vi "SwissSPAD Live_Settings Window.vi"() -> ()   [LabVIEW 2021]
uses:
  SwissSPAD Live_SS2 DAQ Parameters 3.ctl
  SwissSPAD Live_SS2 Gate Definition.ctl
  SwissSPAD Live_File Information.ctl
  SwissSPAD Live_Gate Characteristics.ctl
  SwissSPAD Live_Image ROI Information.ctl
  Phasor/Image Binning Options.ctl
  SwissSPAD Live_SSx PCB Version.ctl
  SwissSPAD Live_SS3 DAQ Parameters.ctl
  SwissSPAD Live_SS3 Gate Definition.ctl
  SS3 Gate Width Definition Mode.ctl
  SwissSPAD Live_SS3 Displayed Image v2.ctl
  SwissSPAD Live_Image Display Options.ctl
  SwissSPAD Live_FPGA Data to Display.ctl
  SwissSPAD Live_Settings Q Element.ctl
  SwissSPAD Live_Settings Q Action.ctl
  SwissSPAD Live_Gate Configuration Action.ctl
  SwissSPAD Live_Settings List.ctl
  SwissSPAD Live_SS2 Gate Configuration.ctl
  SwissSPAD Live_Q [Element].ctl
  SwissSPAD Live_Q Event List.ctl
  SwissSPAD Live_Globals.vi
  Variant/Variant to Data/Variant to Data.lvlib
panel:
  in  "Tab Control":T1(tab)
  in  "Top Half":bool
  in  "Bottom Half":bool
  out "Top Connected":bool caption="Connected"
  in  "Connect to Top FPGA":bool
  out "Top FPGA Serial Number":string
  out "Top Bitstream Version":string
  in  "Top Bitfile Path":path
  out "Bottom Connected":bool caption="Connected"
  in  "Connect to FPGA(s)":bool
  out "Detector PCB Version":T2
  out "Bottom FPGA Serial Number":string
  out "Bottom Bitstream Version":string
  in  "Bottom Bitfile Path":path
  in  "Auto Reset FPGA":bool
  in  "Microlens":bool
  in  "SS3 DAQ Parameters":T3={"10 bits"=FALSE, "# Exposure Sequences"=0, "# 1-bit Frame per Gate"=255, "Gate Shift"=0, "# Gate Pairs per Set"=0, "# Sets"=1, "Laser Period"=0.0, "Sync Period"=0.0, "Gate Offset"=0, "Auto-adjust Gate Offset"=FALSE, "Gate Definition"={"gs_psincdec_0"=0, "gs_psincdec_1"=0, "gs_no_shift_adj_1"=0, "gate_adj_2"=0}, "Gate Width (ns)"=0.0, "Reversed Shift"=FALSE, "Intensity Mode"=FALSE, "Gate Definition Mode"=enum."Item 0"} {"Gate Width (ns)" min=0.0 max=100.0 format="%#_5g"; "# Sets" min=1}
  in  "Buffer Size (# 8-bit Gates)":u32=1 min=1
  out "Gate Characteristics":T6 {"Gate Images Span" format="%#.3g"; "Gate Shift" format="%#.3g"; "Gate Image Exposure" format="%#.3g"; "Gate Image Integration" format="%#.3g"; "Predicted Gate Width" format="%#.3g"}
  in  "Preset Configuration":u16(ring) items=["User-defined configuration", "Gate Configuration 1", "Gate Configuration 2", "Gate Configuration 3", "Gate Configuration 4", "Gate Configuration 5", "Gate Configuration 6", "Gate Configuration 7"]
  in  "SS2 DAQ Parameters":T7={"10 bits"=FALSE, "# Exposure Sequences"=1, "# 1-bit Frame per Gate"=255, "Gate Shift"=0, "# Gates per Set"=1, "# Sets"=1, "Laser Period"=0.0, "Sync Period"=0.0, "Gate Offset"=0, "Auto-adjust Gate Offset"=FALSE, "Gate Definition"={"gs_psincdec_0"=0, "gs_psincdec_1"=0, "gs_psincdec_2"=0, "gs_psincdec_3"=0, "gs_no_shift_adj_1"=0, "gs_no_shift_adj_2"=0, "gs_no_shift_adj_3"=0}, "Reversed Shift"=FALSE} {"Sync Period" min=0.0 max=4.294967295 format="%#.3f"; "Laser Period" min=0.0 format="%#.3f"; "# 1-bit Frame per Gate" min=255 max=255; "# Sets" min=1; "# Gates per Set" min=1}
  in  "FPGA Data to Display":T9
  in  "Use Histogram Cursors":bool
  in  "SS3 Displayed Image":T10 caption="Image to Display"
  in  "Image Binning Options":T11={"Use Image Binning"=FALSE, "X Bin"=1, "Y Bin"=1} {"Y Bin" min=1; "X Bin" min=1}
  in  "Image ROI Information":T12
  in  "Image Display Options":T13={"Remove Screamers"=FALSE, "Delta"=0.0, "Equalize Histogram"=FALSE, "Percentile"=2.0, "Hot Pixel Mask Image"=path "", "Use Hot Pixel Mask"=FALSE} {"Percentile" min=0 max=100}
  in  "Save Sum of All Gates Preview":bool
  in  "SS3 Hot Pixel Mismatch Detection":bool
  in  "SS3 Gate Slip Correction":bool
  in  "Delay between Datasets":dbl[unit]
  in  "Scrambled File Flag":bool
  in  "# Datasets in Series":i32=1 min=1
  in  "File Information":T14={"File Folder"=path "", "File Name"="", "File Index"=0, "Author"="", "Sample"="", "Compression"=FALSE, "Compression Level"=9} {"Compression Level" max=9}
  in  "Histogram Bin Size":i32=256 min=1 step=1
  in  "Verbose Saving":bool
  in  "Verbose Settings":bool
  in  "Use Image Display Options":bool
  in  "Histogram Bins Number":i32=256 min=1 step=1
  # "Image Histogram"
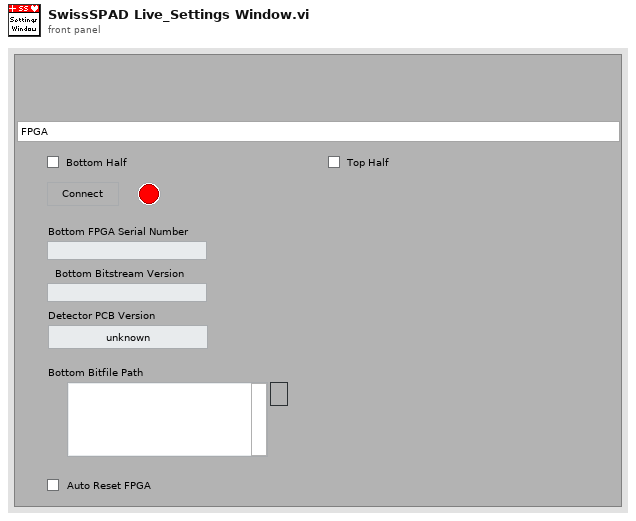
[diagram p1: front panel]
types:
  T1 = enum32{"FPGA", "Acquisition Parameters", "Image Parameters", "File Information", "UI Settings"}
  T2 = typedef "SwissSPAD Live_SSx PCB Version.ctl" = enum16{"unknown", "SS2 PCB1", "SS2 PCB2", "SS3 PCB1"}
  T3 = typedef "SwissSPAD Live_SS3 DAQ Parameters.ctl" = cluster{"10 bits":bool, "# Exposure Sequences":u32, "# 1-bit Frame per Gate":u32, "Gate Shift":u32, "# Gate Pairs per Set":u32, "# Sets":u32, "Laser Period":dbl[unit], "Sync Period":dbl[unit], "Gate Offset":u32, "Auto-adjust Gate Offset":bool, "Gate Definition":T4, "Gate Width (ns)":dbl, "Reversed Shift":bool, "Intensity Mode":bool, "Gate Definition Mode":T5}
  T4 = typedef "SwissSPAD Live_SS3 Gate Definition.ctl" = cluster{"gs_psincdec_0":u32, "gs_psincdec_1":u32, "gs_no_shift_adj_1":u32, "gate_adj_2":u32}
  T5 = typedef "SS3 Gate Width Definition Mode.ctl" = enum32{"Item 0", "Item 1"}
  T6 = typedef "SwissSPAD Live_Gate Characteristics.ctl" = cluster{"Predicted Gate Width":dbl[unit], "Gate Image Integration":dbl[unit], "Gate Image Exposure":dbl[unit], "Gate Shift":dbl[unit], "Gate Images Span":dbl[unit]}
  T7 = typedef "SwissSPAD Live_SS2 DAQ Parameters 3.ctl" = cluster{"10 bits":bool, "# Exposure Sequences":u32, "# 1-bit Frame per Gate":u32, "Gate Shift":u32, "# Gates per Set":u32, "# Sets":u32, "Laser Period":dbl[unit], "Sync Period":dbl[unit], "Gate Offset":u32, "Auto-adjust Gate Offset":bool, "Gate Definition":T8, "Reversed Shift":bool}
  T8 = typedef "SwissSPAD Live_SS2 Gate Definition.ctl" = cluster{"gs_psincdec_0":u32, "gs_psincdec_1":u32, "gs_psincdec_2":u32, "gs_psincdec_3":u32, "gs_no_shift_adj_1":u32, "gs_no_shift_adj_2":u32, "gs_no_shift_adj_3":u32}
  T9 = typedef "SwissSPAD Live_FPGA Data to Display.ctl" = enum16{"Bottom FPGA", "Top FPGA", "Both"}
  T10 = typedef "SwissSPAD Live_SS3 Displayed Image v2.ctl" = enum16{"G2 Gate", "INT Gate", "INT - G2"}
  T11 = typedef "Image Binning Options.ctl" = cluster{"Use Image Binning":bool, "X Bin":i32, "Y Bin":i32}
  T12 = typedef "SwissSPAD Live_Image ROI Information.ctl" = cluster{"Save ROI Only":bool, "Left":u16, "Top":u16, "Right":u16, "Bottom":u16, "Use Current ROI":bool}
  T13 = typedef "SwissSPAD Live_Image Display Options.ctl" = cluster{"Remove Screamers":bool, "Delta":sgl, "Equalize Histogram":bool, "Percentile":sgl, "Hot Pixel Mask Image":path, "Use Hot Pixel Mask":bool}
  T14 = typedef "SwissSPAD Live_File Information.ctl" = cluster{"File Folder":path, "File Name":string, "File Index":u32, "Author":string, "Sample":string, "Compression":bool, "Compression Level":u8}
  T15 = typedef "SwissSPAD Live_Settings Q Element.ctl" = cluster{"Action":T16, "Data":variant}
  T16 = typedef "SwissSPAD Live_Settings Q Action.ctl" = enum16{"Idle", "Initialization", "Refresh All Parameters", "Store Current Configuration", "Rename Current Configuration", "Delete Current Configuration", "Update Image ROI Information", "Load Hot Pixel Mask Image", "Quit"}
  T17 = cluster{"Connect to FPGA(s)":refnum<vi>, "Bottom Connected":refnum<vi>, "Preset Configuration":refnum<vi>, "SS2 DAQ Parameters":refnum<vi>, "SS3 DAQ Parameters":refnum<vi>, "SS3 Displayed Image":refnum<vi>, "Bottom FPGA Serial Number":refnum<vi>, "Detector PCB Version":refnum<vi>, "SS3 Gate Slip Correction":refnum<vi>, "Scrambled File Flag":refnum<vi>, "Top Connected":refnum<vi>, "Top FPGA Serial Number":refnum<vi>, "SS3 Hot Pixel Mismatch Detection":refnum<vi>}
  T18 = enum32{"Invalid", "Standard", "Closed", "Hidden", "Minimized", "Maximized"}
  T19 = typedef "SwissSPAD Live_Gate Configuration Action.ctl" = enum16{"Get Gate Configuration Name", "Get Configuration by Name", "Add Gate Configuration", "Delete Gate Configuration", "Rename Gate Configuration"}
  T20 = typedef "SwissSPAD Live_Settings List.ctl" = enum16{"FPGA:Bottom Half", "FPGA:Top Half", "FPGA:Bottom Bitfile Path", "FPGA:Top Bitfile Path", "FPGA:Bottom Bitstream Version", "FPGA:Top Bitstream Version", "FPGA:Auto Reset FPGA", "FPGA:Bottom FPGA Serial Number", "FPGA:Top FPGA Serial Number", "FPGA:Detector PCB Version", "Acquisition Parameters:Microlens", "Acquisition Parameters:SS2 DAQ Parameters", "Acquisition Parameters:Gate Configuration Array", "Acquisition Parameters:SS3 DAQ Parameters", "Acquisition Parameters:Buffer Size (# 8-bit Gates)", "File Information:File Information", "File Information:# Datasets in Series", "File Information:Scrambled File Flag", "File Information:SS3 Gate Slip Correction", "File Information:SS3 Hot Pixel Mismatch Detection", "File Information:Delay between Datasets", "File Information:Save Sum of All Gates Preview", "Image Parameters:Image ROI Information", "Image Parameters:Image Binning Options", "Image Parameters:SS3 Displayed Image", "Image Parameters:Image Display Options", "Image Parameters:Use Histogram Cursors", "Image Parameter:FPGA Data to Display", "UI Settings:Histogram Bins Number", "UI Settings:Histogram Bin Size", "UI Settings:Use Image Display Options", "UI Settings:Verbose Settings", "UI Settings:Verbose Saving"}
  T21 = typedef "SwissSPAD Live_Internal Variables.ctl" = cluster{"okCFrontPanelDevices Refnum":refnum<k24>, "Bottom Device Refnum":refnum<k24>, "Display Image":T22, "# Live Images":i32, "relative s":dbl, "# Image Sets":i32, "Message":string, "Current Image Set":i32, "# Datasets in Series":i32, "Current Dataset":i32, "Live Mode":bool, "Recording Mode":bool, "Record Button":refnum<vi>, "\nLive Button":refnum<vi>, "SwissSPAD Live Gate Image Data Q Name":string, "Discard First Image":bool, "Image Information":T12, "Image Binning Options":T11, "Bottom FPGA Serial Number":string, "Detector PCB Version":T2, "# Acquisitions":u32, "10 bits":bool, "Top FPGA Serial Number":string, "Top Device Refnum":refnum<k24>, "okCFrontPanel Refnum":refnum<k24>}
  T22 = typedef "IMAQ Image.ctl" = refnum<image>
  T23 = typedef "SwissSPAD Live_SS2 Gate Configuration.ctl" = cluster{"Gate Configuration":string, "Gate Offset":u32, "Gate Definition":T8}
  T24 = typedef "SwissSPAD Live_Q [Element].ctl" = cluster{"SwissSPAD Q Event":T25, "Data":variant}
  T25 = typedef "SwissSPAD Live_Q Event List.ctl" = enum16{"---- UI ----", "Idle", "Initialization", "Init FPGA(s)", "Init Top FPGA (deprecated)", "FPGA(s) Status", "Top FPGA Status (deprecated)", "Reset FPGA(s)", "Reset Top FPGA (deprecated)", "Refresh Display Image", "Quit", "---- DAQ ----", "Start Recording", "Start Live Acquisition", "Initialize Recording Mode", "Initialize FPGA (Live Mode)", "Get Image Set", "Get Single Image", "Update Image Display", "Stop Live Acquisition", "Stop Data Recording", "Stop Data Saving", "---- Image ----", "Copy Data to Clipboard", "Set Image Palette", "Save Displayed Image with Overlay", "Save Image Data as TIFF"}
  T26 = typedef "SS2 DAQ_Settings Window Messages.ctl" = enum16{"Idle", "Subscribe", "Unsubscribe", "Refresh Parameter", "Refresh All Parameters", "Quit"}
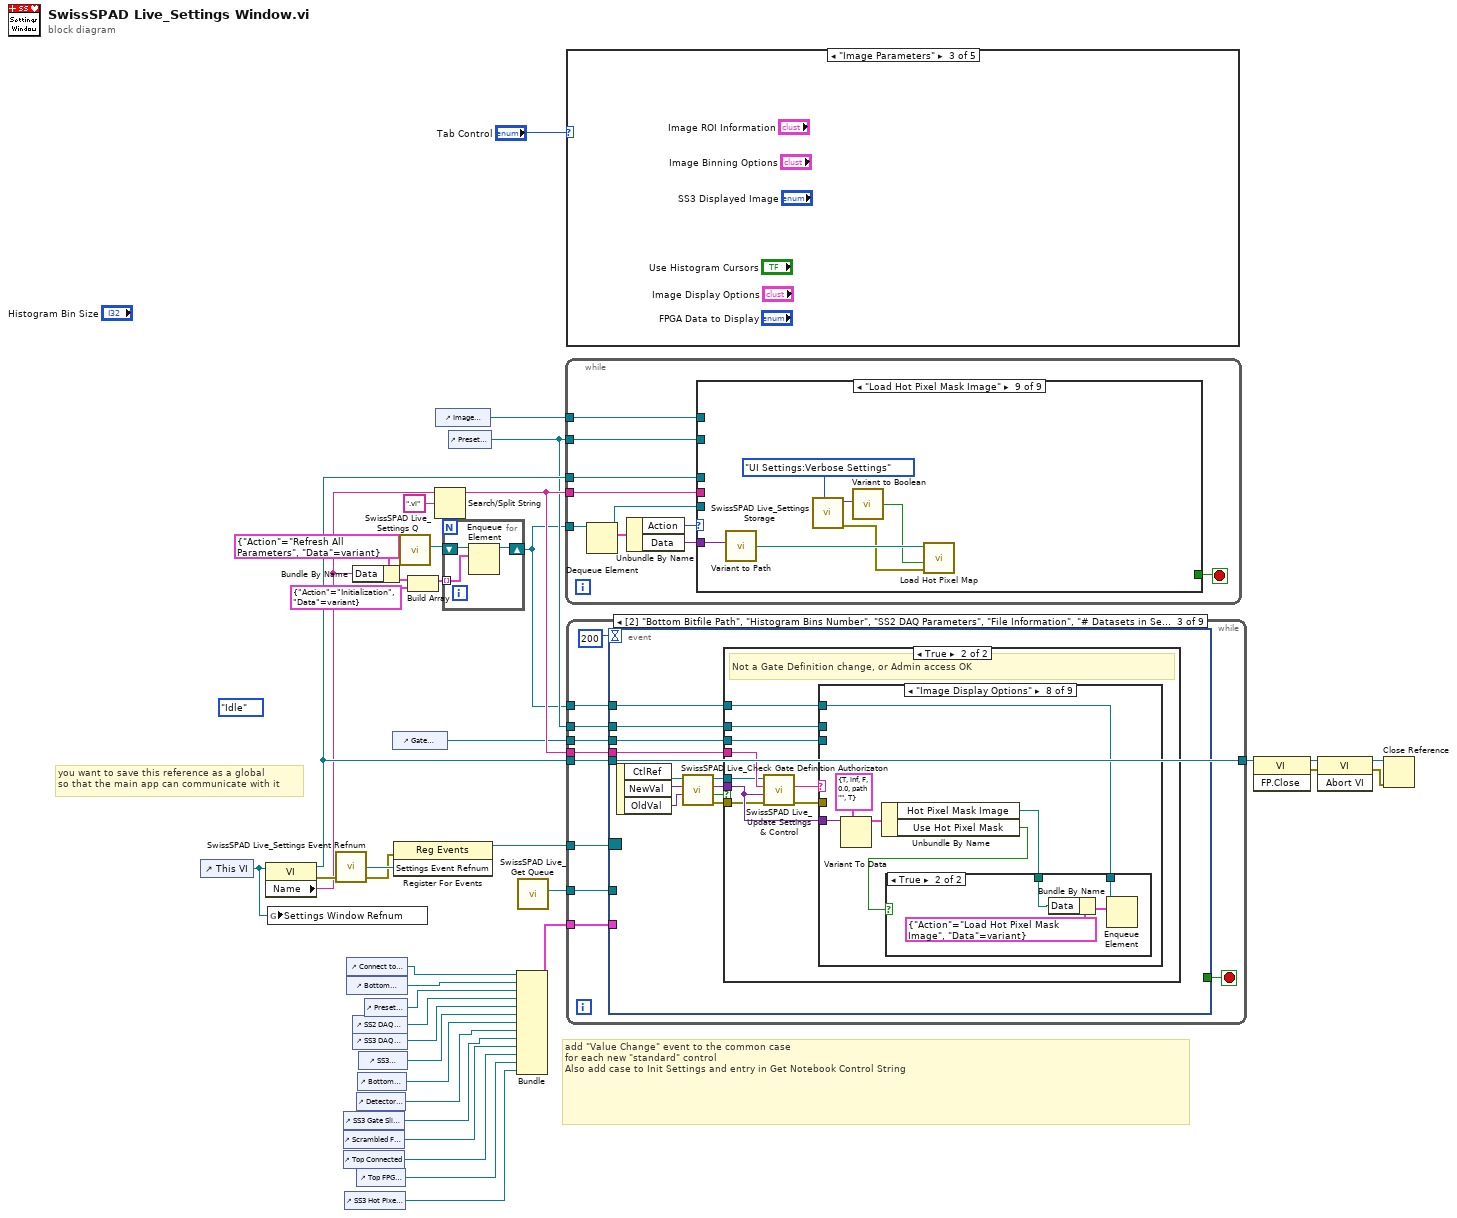
[diagram p0: block diagram]
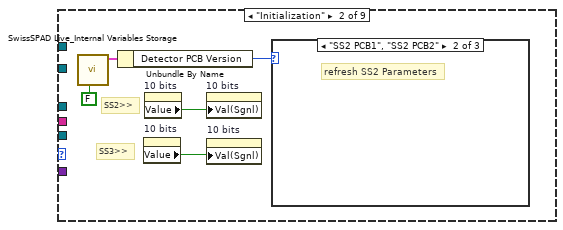
[diagram p3: hidden frame]
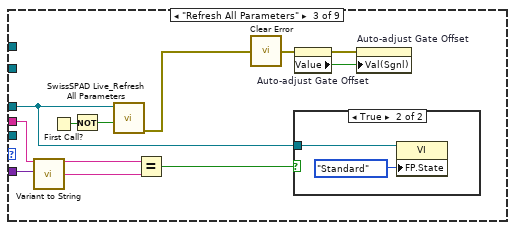
[diagram p6: hidden frame]
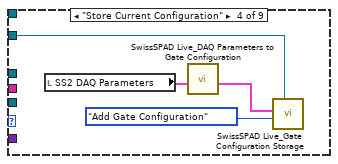
[diagram p8: hidden frame]
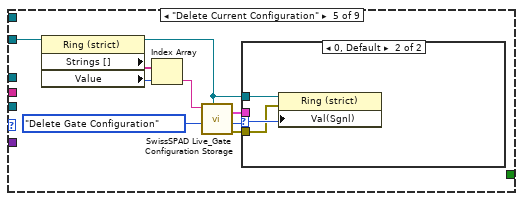
[diagram p9: hidden frame]
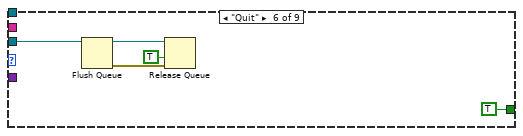
[diagram p11: hidden frame]
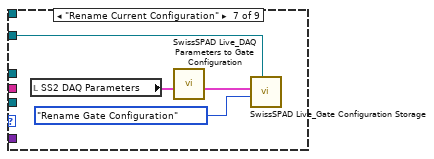
[diagram p12: hidden frame]
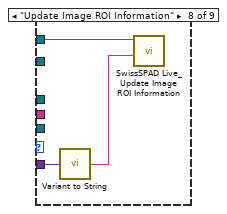
[diagram p13: hidden frame]
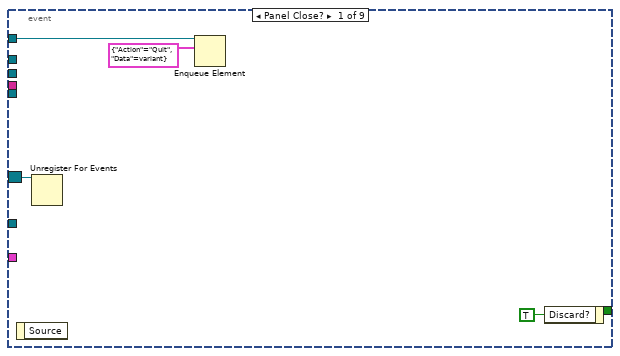
[diagram p14: hidden frame]
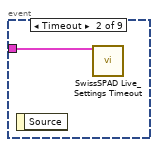
[diagram p15: hidden frame]
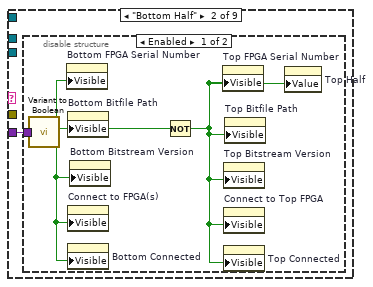
[diagram p18: hidden frame]
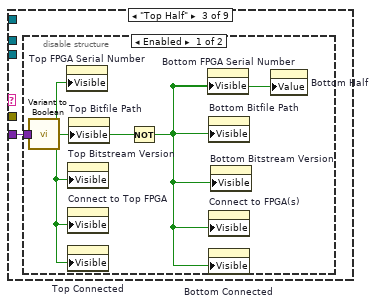
[diagram p20: hidden frame]
diagram:
  (unwired) SwissSPAD_Live_Settings_Q_Action."Idle" ("Action")
  # "you want to save this reference as a global\nso that the main app can communicate with it"
  # "add \"Value Change\" event to the common case\nfor each new \"standard\" control\nAlso add case to Init Settings and entry in Get Notebook Control String"
  n1 = control-ref of="This VI"() -> (w29:refnum<vi>)
  n2 = property class="VI"(reference=w29) -> (reference out=w30:refnum<vi>, error out=w35:errorcluster, "Name"=w9:string)  [unwired: 1 in]
  n3 = global write "SwissSPAD Live_Globals.vi" "Settings Window Refnum"(w29) -> ()
  n4 = call "SwissSPAD Live_Settings Event Refnum.vi"("Error In"=w35) -> ("Settings Event Refnum"=w39:refnum<user-event>, "Error Out"=w38:errorcluster)  [unwired: 7 in]
  n5 = control-ref of="SS3 Gate Slip Correction"() -> (w8:refnum<vi>)
  n6 = control-ref of="Scrambled File Flag"() -> (w7:refnum<vi>)
  n7 = control-ref of="Top Connected"() -> (w6:refnum<vi>)
  n8 = control-ref of="SS3 Hot Pixel Mismatch Detection"() -> (w4:refnum<vi>)
  n9 = control-ref of="Connect to FPGA(s)"() -> (w23:refnum<vi>)
  n10 = control-ref of="Bottom Connected"() -> (w22:refnum<vi>)
  n11 = Bundle By Name(cluster=T15 {"Action"=enum."Refresh All Parameters", "Data"=variant} ("element"), "Data"=w9) -> (w11:T15)
  n12 = control-ref of="SS2 DAQ Parameters"() -> (w20:refnum<vi>)
  n13 = control-ref of="SS3 DAQ Parameters"() -> (w19:refnum<vi>)
  n14 = control-ref of="Detector PCB Version"() -> (w15:refnum<vi>)
  n15 = control-ref of="Top FPGA Serial Number"() -> (w5:refnum<vi>)
  n16 = control-ref of="Bottom FPGA Serial Number"() -> (w16:refnum<vi>)
  n17 = control-ref of="SS3 Displayed Image"() -> (w18:refnum<vi>)
  n18 = control-ref of="Preset Configuration"() -> (w21:refnum<vi>)
  n19 = control-ref of="Gate Characteristics"() -> (w25:refnum<vi>)
  n20 = register-events(error in=w38, w39) -> (reference out=w36:refnum<event-registration>)  [unwired: 1 in, 1 out]
  n21 = call "SwissSPAD Live_Settings Q.vi"() -> ("Queue out"=w26:refnum<queue>)  [unwired: 10 in, 1 out]
  n22 = Build Array(w11, T15 {"Action"=enum."Initialization", "Data"=variant} ("element")) -> (w12:T15[])
  n23 = Search/Split String(string=w9, search string/char (-)=".vi") -> (substring before match=w32:string)  [unwired: 1 in, 2 out]
  n24 = control-ref of="Image Information"() -> (w27:refnum<vi>)
  n25 = for {
    tunnel: w12 -> [w40] mode=indexing
    shift-right: [w41] -> w14
    shift-left: w26 -> [w42]
    n26 = Enqueue Element(queue=w42, element=w40) -> (queue out=w41:refnum<queue>)  [unwired: 2 in, 2 out]
  }
  n27 = control-ref of="Preset Configuration"() -> (w28:refnum<vi>)
  n28 = Bundle("Connect to FPGA(s)"=w23, "Bottom Connected"=w22, "Preset Configuration"=w21, "SS2 DAQ Parameters"=w20, "SS3 DAQ Parameters"=w19, "SS3 Displayed Image"=w18, "Bottom FPGA Serial Number"=w16, "Detector PCB Version"=w15, "SS3 Gate Slip Correction"=w8, "Scrambled File Flag"=w7, "Top Connected"=w6, "Top FPGA Serial Number"=w5, "SS3 Hot Pixel Mismatch Detection"=w4) -> (w17:T17)  [unwired: 1 in]
  n29 = call "SwissSPAD Live_Get Queue.vi"() -> ("SwissSPAD Queue"=w24:refnum<queue>)  [unwired: 10 in, 1 out]
  n30 = while {
    tunnel: w14 -> [w52]
    tunnel: w32 -> [w47]
    tunnel: w30 -> [w46]
    tunnel: w28 -> [w45]
    tunnel: w27 -> [w44]
    stop <- w49 stop-if-true
    n31 = Dequeue Element(queue=w52) -> (queue out=w43:refnum<queue>, element=w51:T15)  [unwired: 2 in, 2 out]
    n32 = Unbundle By Name(w51) -> ("Action"=w50:T16, "Data"=w48:variant)
    n33 = case shown="\"Load Hot Pixel Mask Image\"" w50 {
      tunnel: [_ _ _ _ _ TRUE _ _ _] -> w49
      tunnel: w48 -> [_ _ w63 _ _ _ _ w97 w104]
      tunnel: w47 -> [_ _ w64 _ _ _ _ _ _]
      tunnel: w46 -> [_ _ w65 _ _ _ _ _ _]
      tunnel: w45 -> [_ _ _ w71 w82 _ w92 _ _]
      tunnel: w44 -> [_ _ _ _ _ _ _ w98 _]
      tunnel: w43 -> [_ _ _ _ _ w90 _ _ _]
      frame "Idle", Default {
      }
      frame "Initialization" {
        # "SS2>>"
        # "SS3>>"
        n34 = call "SwissSPAD Live_Internal Variables Storage.vi"("Set/Get(F)"=FALSE) -> ("SwissSPAD Live Internal Variables"=w57:T21)  [unwired: 9 in, 1 out]
        n35 = Unbundle By Name(w57) -> ("Detector PCB Version"=w56:T2)
        n36 = property on="10 bits" class="Bool (strict)"() -> ("Value"=w53:bool)  [unwired: 2 in, 2 out]
        n37 = property on="10 bits" class="Bool (strict)"() -> ("Value"=w54:bool)  [unwired: 2 in, 2 out]
        n38 = property on="10 bits" class="Bool (strict)"("Val(Sgnl)"=w54) -> ()  [unwired: 2 in, 2 out]
        n39 = property on="10 bits" class="Bool (strict)"("Val(Sgnl)"=w53) -> ()  [unwired: 2 in, 2 out]
        n40 = case shown="\"SS2 PCB1\", \"SS2 PCB2\"" w56 {
          frame "unknown", Default {
          }
          frame "SS2 PCB1", "SS2 PCB2" {
            # "refresh SS2 Parameters"
          }
          frame "SS3 PCB1" {
            # "refresh SS3 Parameters"
          }
        }
      }
      frame "Refresh All Parameters" {
        n41 = call "Variant to String.vi"("Variant"=w63) -> ("String"=w62:string)  [unwired: 8 in]
        n42 = First Call?() -> (First Call?: T/F=w67:bool)
        n43 = Not(x=w67) -> (.not. x?=w68:bool)
        n44 = call "SwissSPAD Live_Refresh All Parameters.vi"("Verbose (T)"=w68, "VI Refnum in"=w65) -> ("Error Out"=w58:errorcluster)  [unwired: 9 in]
        n45 = Equal?(x=w64, y=w62) -> (x = y?=w66:bool)
        n46 = call "Clear Error.vi"("Error In"=w58) -> ("no Error Out"=w61:errorcluster)  [unwired: 8 in]
        n47 = case shown="True" w66 {
          tunnel: w65 -> [_ w70]
          frame False {
          }
          frame True {
            n48 = property class="VI"(reference=w70, "FP.State"=T18."Standard" ("State")) -> ()  [unwired: 1 in, 2 out]
          }
        }
        n49 = property on="Auto-adjust Gate Offset" class="Bool (strict)"(error in=w61) -> (error out=w59:errorcluster, "Value"=w60:bool)  [unwired: 1 in, 1 out]
        n50 = property on="Auto-adjust Gate Offset" class="Bool (strict)"(error in=w59, "Val(Sgnl)"=w60) -> ()  [unwired: 1 in, 2 out]
      }
      frame "Store Current Configuration" {
        n51 = local read "SS2 DAQ Parameters"() -> (w73:T7)
        n52 = call "SwissSPAD Live_DAQ Parameters to Gate Configuration.vi"("SS2 DAQ Parameters"=w73) -> ("Gate Configuration Definition out"=w72:T23)  [unwired: 10 in]
        n53 = call "SwissSPAD Live_Gate Configuration Storage.vi"("Preset Configuration Refnum"=w71, "Action"=SwissSPAD_Live_Gate_Configuration_Action."Add Gate Configuration", "Gate Configuration Definition in"=w72) -> ()  [unwired: 3 in, 6 out]
      }
      frame "Delete Current Configuration" {
        n54 = property class="Ring (strict)"(reference=w82) -> (reference out=w76:refnum<vi>, "Strings []"=w81:string[], "Value"=w80:u16)  [unwired: 1 in, 1 out]
        n55 = Index Array(array=w81, index=w80) -> (element=w79:string)
        n56 = call "SwissSPAD Live_Gate Configuration Storage.vi"("Preset Configuration Refnum"=w76, "Action"=SwissSPAD_Live_Gate_Configuration_Action."Delete Gate Configuration", "Gate Configuration Name in"=w79) -> ("Error Out"=w75:errorcluster, "Configuration ID"=w78:i32, "Gate Configuration Definition out"=w77:T23)  [unwired: 3 in, 3 out]
        n57 = case shown="0, Default" w78 {
          selector: w78 -> [_ w86]
          tunnel: w77 -> [_ _]
          tunnel: w76 -> [_ w85]
          tunnel: w75 -> [_ w84]
          frame -1 {
          }
          frame 0, Default {
            n58 = property class="Ring (strict)"(reference=w85, error in=w84, "Val(Sgnl)"=w86) -> ()  [unwired: 2 out]
          }
        }
      }
      frame "Quit" {
        n59 = Flush Queue(queue=w90) -> (queue out=w89:refnum<queue>, error out=w87:errorcluster)  [unwired: 1 in, 1 out]
        n60 = Release Queue(queue=w89, force destroy? (F)=TRUE, error in (no error)=w87) -> ()  [unwired: 3 out]
      }
      frame "Rename Current Configuration" {
        n61 = local read "SS2 DAQ Parameters"() -> (w94:T7)
        n62 = call "SwissSPAD Live_DAQ Parameters to Gate Configuration.vi"("SS2 DAQ Parameters"=w94) -> ("Gate Configuration Definition out"=w93:T23)  [unwired: 10 in]
        n63 = call "SwissSPAD Live_Gate Configuration Storage.vi"("Preset Configuration Refnum"=w92, "Action"=SwissSPAD_Live_Gate_Configuration_Action."Rename Gate Configuration", "Gate Configuration Definition in"=w93) -> ()  [unwired: 3 in, 6 out]
      }
      frame "Update Image ROI Information" {
        n64 = call "Variant to String.vi"("Variant"=w97) -> ("String"=w96:string)  [unwired: 8 in]
        n65 = call "SwissSPAD Live_Update Image ROI Information.vi"("Element Changed"=w96, "Image Information Refnum"=w98) -> ()  [unwired: 8 in, 2 out]
      }
      frame "Load Hot Pixel Mask Image" {
        n66 = call "Variant to Path.vi"("Variant"=w104) -> ("Path"=w103:path)  [unwired: 8 in]
        n67 = call "SwissSPAD Live_Settings Storage.vi"("Settings List"=SwissSPAD_Live_Settings_List."UI Settings:Verbose Settings") -> ("Error Out"=w102:errorcluster, "Variant Data out"=w100:variant)  [unwired: 9 in]
        n68 = call "Variant to Boolean.vi"("Variant"=w100) -> ("Value"=w99:bool)  [unwired: 8 in]
        n69 = call "Load Hot Pixel Map.vi"("Error In"=w102, "Verbose (F)"=w99, "Hot Pixel Mask Image Path"=w103) -> ()  [unwired: 7 in, 2 out]
      }
    }
  }
  n70 = case shown="\"Image Parameters\"" "Tab Control" {
    frame "FPGA" {
    }
    frame "Acquisition Parameters" {
    }
    frame "Image Parameters" {
    }
    frame "File Information" {
    }
    frame "UI Settings" {
    }
  }
  n71 = while {
    tunnel: w30 -> [w112]
    tunnel: [w112] -> w37
    tunnel: w36 -> [w113]
    tunnel: w32 -> [w111]
    tunnel: w14 -> [w110]
    tunnel: w28 -> [w109]
    tunnel: w25 -> [w108]
    tunnel: w24 -> [w106]
    tunnel: w17 -> [w105]
    stop <- w114 stop-if-true
    n72 = event shown="[2] \"Bottom Bitfile Path\", \"Histogram Bins Number\", \"SS2 DAQ Parameters\", \"File Information\", \"# Datasets in Series\", \"Buffer Size (# 8-bit Gates)\", \"Image Binning Options\", \"Scrambled File Flag\", \"Auto Reset FPGA\", \"Delay between Datasets\", \"SS3 DAQ Parameters\", \"SS3 Displayed Image\", \"Top Bitfile Path\", \"Top Connected\", \"Bottom Connected\", \"Bottom Half\", \"Top Half\", \"SS3 Gate Slip Correction\", \"Image Display Options\", \"Use Image Display Options\", \"FPGA Data to Display\", \"Microlens\", \"Verbose Settings\", \"Verbose Saving\", \"SS3 Hot Pixel Mismatch Detection\", \"Save Sum of All Gates Preview\", \"Use Histogram Cursors\", \"Histogram Bin Size\": Value Change" {
      selector: w113 -> [w117 _ _ _ _ _ w231 _ _]
      dyn-events: _ -> [_ _ _ _ _ _ _ _ _]
      timeout: 200 -> [_ _ _ _ _ _ _ _ _]
      tunnel: [w118 _ _ _ _ _ w233 _ _] -> w114
      tunnel: w112 -> [_ _ _ _ _ _ w236 _ _]
      tunnel: w111 -> [_ _ w129 _ w206 _ w234 _ _]
      tunnel: w110 -> [w116 _ w121 w204 _ w227 w232 _ _]
      tunnel: w109 -> [_ _ w127 _ w209 _ _ _ _]
      tunnel: w108 -> [_ _ w123 _ w208 _ _ _ _]
      tunnel: w106 -> [_ _ _ _ _ _ _ w266 w284]
      tunnel: w105 -> [_ w119 _ _ w205 _ _ _ _]
      event Panel Close? {
        w118 = TRUE ("Discard?")
        n73 = event-data() -> ()  [unwired: 1 in, 1 out]
        n74 = Unregister For Events(event registration refnum=w117) -> ()  [unwired: 1 in, 1 out]
        n75 = Enqueue Element(queue=w116, element=T15 {"Action"=enum."Quit", "Data"=variant}) -> ()  [unwired: 2 in, 3 out]
        n76 = event-data("Discard?"=w118) -> ()  [unwired: 1 in, 1 out]
      }
      event Timeout {
        n77 = event-data() -> ()  [unwired: 1 in, 1 out]
        n78 = call "SwissSPAD Live_Settings Timeout.vi"("Settings Control Refnums"=w119) -> ()  [unwired: 10 in, 1 out]
      }
      event "Bottom Bitfile Path", "Histogram Bins Number", "# Datasets in Series", "Buffer Size (# 8-bit Gates)", "Scrambled File Flag", "Auto Reset FPGA", "Delay between Datasets", "Top Bitfile Path", "Top Connected", "Bottom Connected", "Bottom Half", "Top Half", "SS3 Gate Slip Correction", "Use Image Display Options", "Microlens", "Verbose Settings", "Verbose Saving", "SS3 Hot Pixel Mismatch Detection", "Save Sum of All Gates Preview", "Use Histogram Cursors", "Histogram Bin Size": Value Change {
        n79 = event-data() -> ("CtlRef"=w130:refnum<vi>, "NewVal"=w128:variant, "OldVal"=w120:variant)  [unwired: 1 in]
        n80 = call "SwissSPAD Live_Check Gate Definition Authorizaton.vi"("OldVal"=w120, "NewVal"=w128, "Control Refnum"=w130) -> ("Error Out"=w122:errorcluster, "Change Accepted?"=w124:bool, "NewVal"=w125:variant, "Control Refnum"=w126:refnum<vi>)  [unwired: 5 in]
        n81 = case shown="True" w124 {
          tunnel: w129 -> [_ w139]
          tunnel: w127 -> [_ w136]
          tunnel: w126 -> [_ w135]
          tunnel: w125 -> [_ w134]
          tunnel: w123 -> [_ w133]
          tunnel: w122 -> [_ w132]
          tunnel: w121 -> [_ w131]
          frame False {
            # "Not admin & Gate Definition change cancelled"
          }
          frame True {
            # "Not a Gate Definition change, or Admin access OK"
            n82 = call "SwissSPAD Live_Update Settings & Control.vi"("Error In"=w132, "Value"=w134, "Sender"=w139, "CtlRef"=w135) -> ("Error Out"=w137:errorcluster, "Control Label"=w138:string)  [unwired: 6 in]
            n83 = case shown="\"Image Display Options\"" w138 {
              tunnel: w134 -> [_ w140 w144 w154 w161 w174 w180 w185 _]
              tunnel: w137 -> [_ _ _ w152 w159 w173 w179 _ _]
              tunnel: w136 -> [_ _ _ _ _ w166 _ _ _]
              tunnel: w133 -> [_ _ _ _ _ w162 w176 _ _]
              tunnel: w131 -> [_ _ _ _ _ _ _ w183 _]
              frame "", Default {
              }
              frame "Bottom Half" {
                n84 = disable-structure shown="Enabled" {
                  disable-tunnel: w140 -> [w143 _]
                  frame Enabled {
                    n85 = call "Variant to Boolean.vi"("Variant"=w143) -> ("Value"=w142:bool)  [unwired: 8 in]
                    n86 = property on="Bottom FPGA Serial Number" class="Str"("Visible"=w142) -> ()  [unwired: 2 in, 2 out]
                    n87 = property on="Bottom Bitfile Path" class="Path"("Visible"=w142) -> ()  [unwired: 2 in, 2 out]
                    n88 = property on="Connect to FPGA(s)" class="Bool"("Visible"=w142) -> ()  [unwired: 2 in, 2 out]
                    n89 = property on="Bottom Connected" class="Bool (strict)"("Visible"=w142) -> ()  [unwired: 2 in, 2 out]
                    n90 = property on="Bottom Bitstream Version" class="Str"("Visible"=w142) -> ()  [unwired: 2 in, 2 out]
                    n91 = Not(x=w142) -> (.not. x?=w141:bool)
                    n92 = property on="Top FPGA Serial Number" class="Str"("Visible"=w141) -> ()  [unwired: 2 in, 2 out]
                    n93 = property on="Top Bitstream Version" class="Str"("Visible"=w141) -> ()  [unwired: 2 in, 2 out]
                    n94 = property on="Connect to Top FPGA" class="Bool"("Visible"=w141) -> ()  [unwired: 2 in, 2 out]
                    n95 = property on="Top Connected" class="Bool (strict)"("Visible"=w141) -> ()  [unwired: 2 in, 2 out]
                    n96 = property on="Top Bitfile Path" class="Path"("Visible"=w141) -> ()  [unwired: 2 in, 2 out]
                    n97 = property on="Top Half" class="Bool (strict)"("Value"=w141) -> ()  [unwired: 2 in, 2 out]
                  }
                  frame Disabled {
                  }
                }
              }
              frame "Top Half" {
                n98 = disable-structure shown="Enabled" {
                  disable-tunnel: w144 -> [w147 _]
                  frame Enabled {
                    n99 = call "Variant to Boolean.vi"("Variant"=w147) -> ("Value"=w146:bool)  [unwired: 8 in]
                    n100 = property on="Top FPGA Serial Number" class="Str"("Visible"=w146) -> ()  [unwired: 2 in, 2 out]
                    n101 = property on="Top Bitstream Version" class="Str"("Visible"=w146) -> ()  [unwired: 2 in, 2 out]
                    n102 = property on="Connect to Top FPGA" class="Bool"("Visible"=w146) -> ()  [unwired: 2 in, 2 out]
                    n103 = property on="Top Connected" class="Bool (strict)"("Visible"=w146) -> ()  [unwired: 2 in, 2 out]
                    n104 = property on="Top Bitfile Path" class="Path"("Visible"=w146) -> ()  [unwired: 2 in, 2 out]
                    n105 = Not(x=w146) -> (.not. x?=w145:bool)
                    n106 = property on="Bottom FPGA Serial Number" class="Str"("Visible"=w145) -> ()  [unwired: 2 in, 2 out]
                    n107 = property on="Bottom Bitfile Path" class="Path"("Visible"=w145) -> ()  [unwired: 2 in, 2 out]
                    n108 = property on="Connect to FPGA(s)" class="Bool"("Visible"=w145) -> ()  [unwired: 2 in, 2 out]
                    n109 = property on="Bottom Connected" class="Bool (strict)"("Visible"=w145) -> ()  [unwired: 2 in, 2 out]
                    n110 = property on="Bottom Bitstream Version" class="Str"("Visible"=w145) -> ()  [unwired: 2 in, 2 out]
                    n111 = property on="Bottom Half" class="Bool (strict)"("Value"=w145) -> ()  [unwired: 2 in, 2 out]
                  }
                  frame Disabled {
                  }
                }
              }
              frame "Bottom Bitfile Path" {
                n112 = call "Variant to Path.vi"("Variant"=w154) -> ("Path"=w153:path)  [unwired: 8 in]
                n113 = call "SwissSPAD Live_Bitfile Version.vi"("error in (no error)"=w152, "Bitfile Path"=w153) -> ("error out"=w151:errorcluster, "Bitfile Version"=w148:string)  [unwired: 8 in]
                n114 = property on="Bottom Bitstream Version" class="Str"(error in=w151, "Value"=w148) -> (error out=w150:errorcluster)  [unwired: 1 in, 1 out]
                n115 = call "SwissSPAD Live_Settings Storage.vi"("Settings List"=SwissSPAD_Live_Settings_List."FPGA:Bottom Bitstream Version", "Error In"=w150, "Variant Data in"=w148) -> ()  [unwired: 7 in, 2 out]
              }
              frame "Top Bitfile Path" {
                n116 = call "Variant to Path.vi"("Variant"=w161) -> ("Path"=w160:path)  [unwired: 8 in]
                n117 = call "SwissSPAD Live_Bitfile Version.vi"("error in (no error)"=w159, "Bitfile Path"=w160) -> ("error out"=w158:errorcluster, "Bitfile Version"=w155:string)  [unwired: 8 in]
                n118 = property on="Top Bitstream Version" class="Str"(error in=w158, "Value"=w155) -> (error out=w157:errorcluster)  [unwired: 1 in, 1 out]
                n119 = call "SwissSPAD Live_Settings Storage.vi"("Settings List"=SwissSPAD_Live_Settings_List."FPGA:Top Bitstream Version", "Error In"=w157, "Variant Data in"=w155) -> ()  [unwired: 7 in, 2 out]
              }
              frame "SS2 DAQ Parameters" {
                n120 = Variant To Data(error in=w173, type=T7 {"10 bits"=FALSE, "# Exposure Sequences"=0, "# 1-bit Frame per Gate"=255, "Gate Shift"=0, "# Gates per Set"=0, "# Sets"=1, "Laser Period"=0.0, "Sync Period"=0.0, "Gate Offset"=0, "Auto-adjust Gate Offset"=FALSE, "Gate Definition"={"gs_psincdec_0"=0, "gs_psincdec_1"=0, "gs_psincdec_2"=0, "gs_psincdec_3"=0, "gs_no_shift_adj_1"=0, "gs_no_shift_adj_2"=0, "gs_no_shift_adj_3"=0}, "Reversed Shift"=FALSE} ("SS2 DAQ Parameters"), Variant=w174) -> (data=w165:T7, error out=w164:errorcluster)
                n121 = Unbundle By Name(w165) -> ("Gate Definition"=w168:T8, "Gate Offset"=w167:u32)
                n122 = call "SwissSPAD Live_Compute SS2 Gate Characteristics.vi"("Gate Characteristics Refnum"=w162, "Error In"=w164, "SS2 DAQ Parameters"=w165) -> ("Error Out"=w163:errorcluster)  [unwired: 7 in, 1 out]
                n123 = Bundle By Name(cluster=T23 {"Gate Configuration"="", "Gate Offset"=0, "Gate Definition"={"gs_psincdec_0"=0, "gs_psincdec_1"=0, "gs_psincdec_2"=0, "gs_psincdec_3"=0, "gs_no_shift_adj_1"=0, "gs_no_shift_adj_2"=0, "gs_no_shift_adj_3"=0}} ("Gate Configuration Definition in"), "Gate Definition"=w168, "Gate Offset"=w167) -> (w169:T23)
                n124 = call "SwissSPAD Live_Gate Configuration Storage.vi"("Preset Configuration Refnum"=w166, "Error In"=w163, "Action"=SwissSPAD_Live_Gate_Configuration_Action."Get Gate Configuration Name", "Gate Configuration Definition in"=w169) -> ()  [unwired: 2 in, 6 out]
              }
              frame "SS3 DAQ Parameters" {
                n125 = Variant To Data(error in=w179, type=T3 {"10 bits"=FALSE, "# Exposure Sequences"=0, "# 1-bit Frame per Gate"=255, "Gate Shift"=0, "# Gate Pairs per Set"=0, "# Sets"=1, "Laser Period"=0.0, "Sync Period"=0.0, "Gate Offset"=0, "Auto-adjust Gate Offset"=FALSE, "Gate Definition"={"gs_psincdec_0"=0, "gs_psincdec_1"=0, "gs_no_shift_adj_1"=0, "gate_adj_2"=0}, "Gate Width (ns)"=0.0, "Reversed Shift"=FALSE, "Intensity Mode"=FALSE, "Gate Definition Mode"=enum."Item 0"} ("SS3 DAQ Parameters"), Variant=w180) -> (data=w175:T3, error out=w177:errorcluster)
                n126 = call "SwissSPAD Live_Compute SS3 Gate Characteristics.vi"("Gate Characteristics Refnum"=w176, "Error In"=w177, "SS3 DAQ Parameters"=w175) -> ()  [unwired: 7 in, 2 out]
              }
              frame "Image Display Options" {
                n127 = Variant To Data(type=T13 {"Remove Screamers"=TRUE, "Delta"=inf, "Equalize Histogram"=FALSE, "Percentile"=0.0, "Hot Pixel Mask Image"=path "", "Use Hot Pixel Mask"=TRUE} ("Hot Pixel Removal"), Variant=w185) -> (data=w184:T13)  [unwired: 1 in, 1 out]
                n128 = Unbundle By Name(w184) -> ("Hot Pixel Mask Image"=w182:path, "Use Hot Pixel Mask"=w181:bool)
                n129 = case shown="True" w181 {
                  tunnel: w183 -> [_ w190]
                  tunnel: w182 -> [_ w187]
                  frame False {
                  }
                  frame True {
                    n130 = Bundle By Name(cluster=T15 {"Action"=enum."Load Hot Pixel Mask Image", "Data"=variant} ("element"), "Data"=w187) -> (w188:T15)
                    n131 = Enqueue Element(queue=w190, element=w188) -> ()  [unwired: 2 in, 3 out]
                  }
                }
              }
              frame "Background File Path (Live Display)" {
              }
            }
          }
        }
      }
      event Value Change {
        n132 = event-data() -> ("OldVal.Use Current ROI"=w201:bool, "NewVal.Use Current ROI"=w200:bool, "OldVal.Save ROI Only"=w197:bool, "NewVal.Save ROI Only"=w196:bool)  [unwired: 1 in]
        n133 = Not Equal?(x=w201, y=w200) -> (x != y?=w199:bool)
        n134 = Not Equal?(x=w197, y=w196) -> (x != y?=w194:bool)
        n135 = Select(t="Use Current ROI" ("name (unnamed)"), s=w199, f="ROI" ("name (unnamed)")) -> (s? t:f=w193:string)
        n136 = Select(t="Only Save ROI" ("name (unnamed)"), s=w194, f=w193) -> (s? t:f=w191:string)
        n137 = Bundle By Name(cluster=T15 {"Action"=enum."Update Image ROI Information", "Data"=variant} ("element"), "Data"=w191) -> (w202:T15)
        n138 = Enqueue Element(queue=w204, element=w202) -> ()  [unwired: 2 in, 3 out]
      }
      event "Preset Configuration": Value Change {
        n139 = event-data() -> ("NewVal"=w214:u16)  [unwired: 1 in]
        n140 = property on="Preset Configuration" class="Ring (strict)"() -> ("Strings []"=w215:string[])  [unwired: 2 in, 2 out]
        n141 = Index Array(array=w215, index=w214) -> (element=w213:string)
        n142 = call "SwissSPAD Live_Gate Configuration Storage.vi"("Preset Configuration Refnum"=w209, "Action"=SwissSPAD_Live_Gate_Configuration_Action."Get Configuration by Name", "Gate Configuration Name in"=w213) -> ("Error Out"=w207:errorcluster, "Configuration ID"=w211:i32, "Gate Configuration Definition out"=w212:T23)  [unwired: 3 in, 3 out]
        n143 = case shown="0, Default" w211 {
          tunnel: w212 -> [_ w223]
          tunnel: w208 -> [_ w224]
          tunnel: w207 -> [_ w222]
          tunnel: w206 -> [_ w219]
          tunnel: w205 -> [_ w217]
          frame -1 {
          }
          frame 0, Default {
            n144 = Unbundle By Name(w217) -> ("SS2 DAQ Parameters"=w216:refnum<vi>)
            n145 = call "SwissSPAD Live_Update SS2 Gate Definition.vi"("error in (no error)"=w222, "Gate Configuration Definition"=w223, "SS2 DAQ Parameters Refnum"=w216) -> ("error out"=w221:errorcluster, "SS2 DAQ Parameters"=w218:T7)  [unwired: 6 in, 1 out]
            n146 = call "SwissSPAD Live_Compute SS2 Gate Characteristics.vi"("Gate Characteristics Refnum"=w224, "Error In"=w221, "SS2 DAQ Parameters"=w218) -> ("Error Out"=w220:errorcluster)  [unwired: 7 in, 1 out]
            n147 = call "SwissSPAD Live_Update Settings & Control.vi"("Error In"=w220, "Value"=w218, "Sender"=w219, "CtlRef"=w216) -> ()  [unwired: 6 in, 2 out]
          }
        }
      }
      event "Preset Configuration": Shortcut Menu Selection (User) {
        n148 = event-data() -> ("ItemTag"=w226:string)  [unwired: 1 in]
        n149 = case shown="\"Rename Configuration\"" w226 {
          tunnel: [_ T15 {"Action"=enum."Store Current Configuration", "Data"=variant} ("element") T15 {"Action"=enum."Delete Current Configuration", "Data"=variant} ("element") T15 {"Action"=enum."Rename Current Configuration", "Data"=variant} ("element")] -> w225
          frame "", Default {
          }
          frame "Store Configuration" {
          }
          frame "Delete Configuration" {
          }
          frame "Rename Configuration" {
          }
        }
        n150 = Enqueue Element(queue=w227, element=w225) -> ()  [unwired: 2 in, 3 out]
      }
      event User Event {
        n151 = event-data() -> ("Settings Message"=w239:T26, "Control Label"=w238:string, "Data"=w237:variant, "Sender"=w235:string)  [unwired: 1 in]
        n152 = case shown="\"Refresh Parameter\"" w239 {
          tunnel: w238 -> [_ _ w248 _]
          tunnel: w237 -> [_ _ w249 _]
          tunnel: w236 -> [_ _ w250 _]
          tunnel: w235 -> [_ _ w247 w262]
          tunnel: w234 -> [_ _ w246 _]
          tunnel: [_ TRUE ("Discard?") _ _] -> w233
          tunnel: w232 -> [_ w242 w244 w265]
          tunnel: w231 -> [_ w240 _ _]
          frame "Idle", Default {
          }
          frame "Quit" {
            n153 = Unregister For Events(event registration refnum=w240) -> ()  [unwired: 1 in, 1 out]
            n154 = Enqueue Element(queue=w242, element=T15 {"Action"=enum."Quit", "Data"=variant}) -> ()  [unwired: 2 in, 3 out]
          }
          frame "Refresh Parameter" {
            n155 = Equal?(x=w247, y=w246) -> (x = y?=w245:bool)
            n156 = case shown="False" w245 {
              tunnel: w250 -> [w254 _]
              tunnel: w249 -> [w252 _]
              tunnel: w248 -> [w253 _]
              tunnel: w244 -> [w251 _]
              frame False {
                n157 = case shown="\"\", Default" w253 {
                  selector: w253 -> [_ w260]
                  tunnel: w254 -> [_ w261]
                  tunnel: w252 -> [_ w259]
                  tunnel: w251 -> [w258 _]
                  frame "Image Information" {
                    n158 = Bundle By Name(cluster=T15 {"Action"=enum."Update Image ROI Information", "Data"=variant} ("element"), "Data"="Use Current ROI") -> (w256:T15)
                    n159 = Enqueue Element(queue=w258, element=w256) -> ()  [unwired: 2 in, 3 out]
                  }
                  frame "", Default {
                    n160 = call "SwissSPAD Live_Refresh Single Parameter.vi"("Data"=w259, "Control Label"=w260, "VI Ref in"=w261) -> ()  [unwired: 8 in, 1 out]
                  }
                }
              }
              frame True {
              }
            }
          }
          frame "Refresh All Parameters" {
            n161 = Bundle By Name(cluster=T15 {"Action"=enum."Refresh All Parameters", "Data"=variant} ("element"), "Data"=w262) -> (w263:T15)
            n162 = Enqueue Element(queue=w265, element=w263) -> ()  [unwired: 2 in, 3 out]
          }
        }
      }
      event "Connect to FPGA(s)": Value Change {
        n163 = event-data() -> ()  [unwired: 1 in, 1 out]
        n164 = call "SwissSPAD Live_Internal Variables Storage.vi"("Set/Get(F)"=FALSE) -> ("Error Out"=w272:errorcluster, "SwissSPAD Live Internal Variables"=w270:T21)  [unwired: 9 in]
        n165 = Unbundle By Name(w270) -> ("Live Mode"=w269:bool, "Recording Mode"=w268:bool)
        n166 = Compound Arithmetic op=OR(w269, w268) -> (w267:bool)
        n167 = case shown="False" w267 {
          tunnel: w272 -> [_ _]
          tunnel: w270 -> [_ _]
          tunnel: w266 -> [w281 _]
          frame False {
            n168 = disable-structure shown="Disabled" {
              disable-tunnel: [w282 _] -> w276
              frame Disabled {
                n169 = property on="Top Bitfile Path" class="Path"() -> ("Value"=w283:path)  [unwired: 2 in, 2 out]
                n170 = property on="Top Bitfile Path" class="Path"("Val(Sgnl)"=w283) -> (error out=w282:errorcluster)  [unwired: 2 in, 1 out]
              }
              frame Enabled {
              }
            }
            n171 = property on="Bottom Bitfile Path" class="Path"() -> ("Value"=w280:path)  [unwired: 2 in, 2 out]
            n172 = property on="10 bits" class="Bool (strict)"() -> (error out=w275:errorcluster, "Value"=w273:bool)  [unwired: 2 in, 1 out]
            n173 = property on="10 bits" class="Bool (strict)"(error in=w275, "Val(Sgnl)"=w273) -> (error out=w274:errorcluster)  [unwired: 1 in, 1 out]
            n174 = property on="Bottom Bitfile Path" class="Path"("Val(Sgnl)"=w280) -> (error out=w278:errorcluster)  [unwired: 2 in, 1 out]
            n175 = Merge Errors(w278, w276, w274) -> (w277:errorcluster)
            n176 = Enqueue Element(queue=w281, element=T24[] [{"SwissSPAD Q Event"=enum."Init FPGA(s)", "Data"=variant}], error in (no error)=w277) -> ()  [unwired: 1 in, 3 out]
          }
          frame True {
            # "Already connected"
            n177 = call "System Error Sound.vi"() -> ()  [unwired: 27 in, 1 out]
          }
        }
      }
      event "Connect to Top FPGA": Value Change {
        n178 = event-data() -> ()  [unwired: 1 in, 1 out]
        n179 = call "SwissSPAD Live_Internal Variables Storage.vi"("Set/Get(F)"=FALSE) -> ("Error Out"=w290:errorcluster, "SwissSPAD Live Internal Variables"=w288:T21)  [unwired: 9 in]
        n180 = Unbundle By Name(w288) -> ("Live Mode"=w287:bool, "Recording Mode"=w286:bool)
        n181 = Compound Arithmetic op=OR(w287, w286) -> (w285:bool)
        n182 = case shown="False" w285 {
          selector: w285 -> [_ w298]
          tunnel: w290 -> [_ _]
          tunnel: w288 -> [_ _]
          tunnel: w284 -> [w293 _]
          frame False {
            n183 = property on="Top Bitfile Path" class="Path"() -> ("Value"=w292:path)  [unwired: 2 in, 2 out]
            n184 = Empty String/Path?(string/path=w292) -> (empty?=w291:bool)
            n185 = case shown="False" w291 {
              tunnel: w293 -> [w297 _]
              tunnel: w292 -> [w294 _]
              frame False {
                n186 = property on="Top Bitfile Path" class="Path"("Val(Sgnl)"=w294) -> (error out=w295:errorcluster)  [unwired: 2 in, 1 out]
                n187 = Enqueue Element(queue=w297, element=T24[] [{"SwissSPAD Q Event"=enum."Init Top FPGA (deprecated)", "Data"=variant}], error in (no error)=w295) -> ()  [unwired: 1 in, 3 out]
              }
              frame True {
              }
            }
          }
          frame True {
            # "Already connected"
            n188 = property on="Top Connected" class="Bool (strict)"("Value"=w298) -> ()  [unwired: 2 in, 2 out]
          }
        }
      }
    }
  }
  n189 = invoke class="VI" method="FP.Close"(reference=w37) -> (reference out=w33:refnum<vi>, error out=w2:errorcluster)  [unwired: 2 in, 1 out]
  n190 = invoke class="VI" method="Abort VI"(reference=w33, error in=w2) -> (reference out=w3:refnum<vi>, error out=w1:errorcluster)  [unwired: 1 in, 1 out]
  n191 = Close Reference(reference=w3, error in (no error)=w1) -> ()  [unwired: 1 out]
